vi "subVI_ZPID.vi"(5 "I":dbl, 7 "P":dbl, 8 "Cumulative Error In":dbl, 11 "Error In":dbl) -> (0 "Cumulative Error Out":dbl, 3 "Control Signal [V]":dbl)   [LabVIEW 2017]
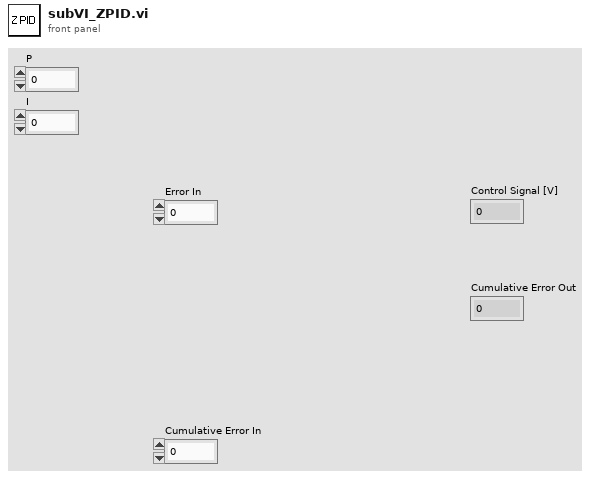
[diagram p1: front panel]
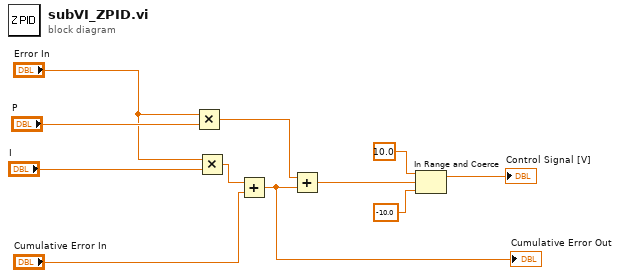
[diagram p0: block diagram]
diagram:
  n1 = Multiply(x="Error In", y="P") -> (x*y=w11:dbl)
  n2 = Multiply(x="Error In", y="I") -> (x*y=w10:dbl)
  n3 = Add(x=w10, y="Cumulative Error In") -> (x+y=w6:dbl)
  "Cumulative Error Out" <- w6
  n4 = Add(x=w11, y=w6) -> (x+y=w5:dbl)
  n5 = In Range and Coerce(upper limit=10.0, x=w5, lower limit=-10.0) -> (coerced(x)=→"Control Signal [V]":dbl)  [unwired: 1 out]
